vi "GetHSL.vi"(0 "ColorHLS in":refnum<class "ColorHSL.lvclass">, 11 "error in (no error)":errorcluster) -> (4 "ColorHLS out":refnum<class "ColorHSL.lvclass">, 6 "H":u8, 8 "S":u8, 10 "L":u8, 15 "error out":errorcluster)   [LabVIEW 2021, in "Picture2D.lvlib" / "ColorHSL.lvclass"]
uses:
  ColorHSL.lvclass
  C:/GitHub/Picture2D/src/Color/Color.lvclass
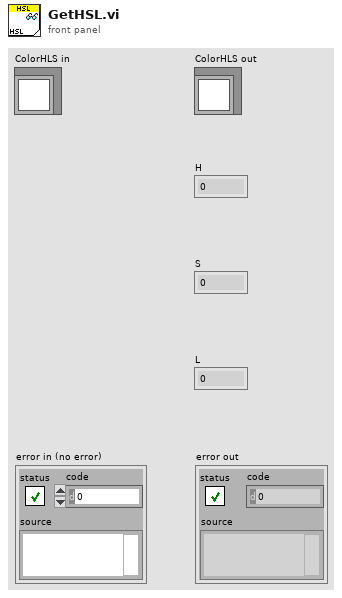
[diagram p1: front panel]
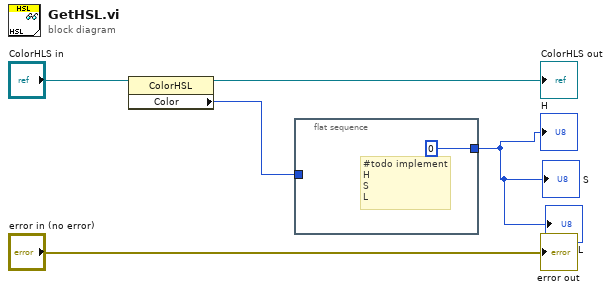
[diagram p0: block diagram]
diagram:
  n1 = property class="ColorHSL"(reference="ColorHLS in") -> (reference out=→"ColorHLS out":refnum<class "ColorHSL.lvclass">, "Color"=w2:u32)  [unwired: 1 in, 1 out]
  n2 = flat-sequence {
    tunnel: w2 -> [_]
    tunnel: [u8 0] -> w1
    frame #0 {
      # "#todo implement\nH\nS\nL"
    }
  }
  "error out" <- "error in (no error)"
  "H" <- w1
  "S" <- w1
  "L" <- w1
